vi "I16toU16.vi"(1 "I16":i16[][](array[numeric])) -> (0 "U16":u16[][](array[numeric]))   [LabVIEW 2015]
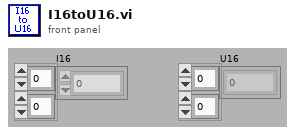
[diagram p1: front panel]
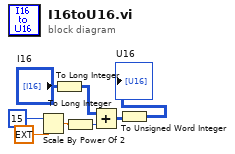
[diagram p0: block diagram]
diagram:
  n1 = Scale By Power Of 2(n=i16 15, x=ext 1.0) -> (x*2^n=w4:ext)
  n2 = To Long Integer(number="I16") -> (32bit integer=w1:i32[][])
  n3 = To Long Integer(number=w4) -> (32bit integer=w8:i32)
  n4 = Add(x=w1, y=w8) -> (x+y=w5:i32[][])
  n5 = To Unsigned Word Integer(number=w5) -> (unsigned 16bit integer=→"U16":u16[][])
